vi "IR AOM word to freq.vi"(0 "Frequency Word In (double)":u64 format="%b") -> (1 "Frequency Out (MHz)":dbl format="%#_6p")   [LabVIEW 2013]
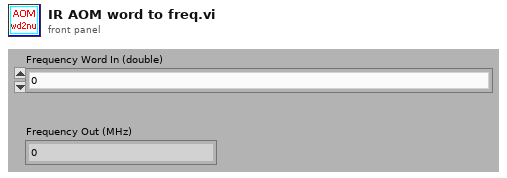
[diagram p1: front panel]
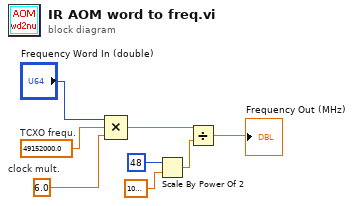
[diagram p0: block diagram]
diagram:
  w6 = 6.0  # clock mult.
  w7 = 49152000.0  # TCXO frequ.
  n1 = Compound Arithmetic op=MULTIPLY("Frequency Word In (double)", w7, w6) -> (w4:dbl)
  n2 = Scale By Power Of 2(n=48, x=1000000.0 ("y")) -> (x*2^n=w2:dbl)
  n3 = Divide(x=w4, y=w2) -> (x/y=→"Frequency Out (MHz)":dbl)
